vi "PumpGilsonGFV.vi"(8 "error in (no error)":errorcluster, 10 "?":T1=enum."Disable Pump", 11 "Variant in":variant) -> (0 "error out":errorcluster, 3 "Variant Out":variant)   [LabVIEW 2013]
doc: "Use this template to build a VI to use as a subVI."
uses:
  General TypeDefs/PumpGilson.ctl
  <vilib>/DAQmx/create/channels.llb/DAQmx Create Channel (DO-Digital Output).vi
  <vilib>/DAQmx/create/channels.llb/DAQmx Create Channel (AO-Voltage-Basic).vi
  <vilib>/DAQmx/write.llb/DAQmx Write (Digital 1D Bool NChan 1Samp 1Line).vi
  <vilib>/DAQmx/write.llb/DAQmx Write (Analog DBL 1Chan 1Samp).vi
  General TypeDefs/PumpGilsonEnum.ctl
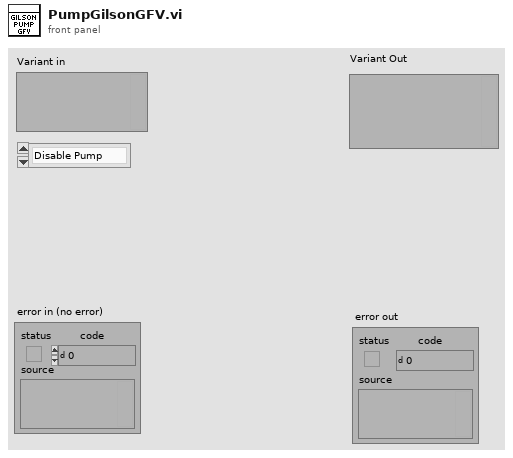
[diagram p1: front panel]
types:
  T1 = typedef "PumpGilsonEnum.ctl" = enum16{"Insert Measuremets Parameters", "Disable Pump", "Enable Pump", "SetPumpState", "SetPumpSpeed", "SetPumpDirection", "GetPumpParameters", "GetCommunicationParameters", "UpdatePumpUI", "ReadFromConfigurationFile", "Init"}
  T2 = typedef "PumpGilson.ctl" = cluster{"Pump Speed Port (analog 0-5 volts)":tag, "Pump State(line 0):Direction(line 1) (TTL output)":tag, "Pump Speed (0-5)":dbl, "Pumping Direction (pull/push)":bool, "Pump State (On/Off)":bool, "Gilson Pump Enabled(On/Off)":bool, "ON time before Acquire (sec)":dbl, "OFF time before Acquire (sec)":dbl}
  T3 = cluster{"ON time before Acquire (sec)":dbl, "OFF time before Acquire (sec)":dbl}
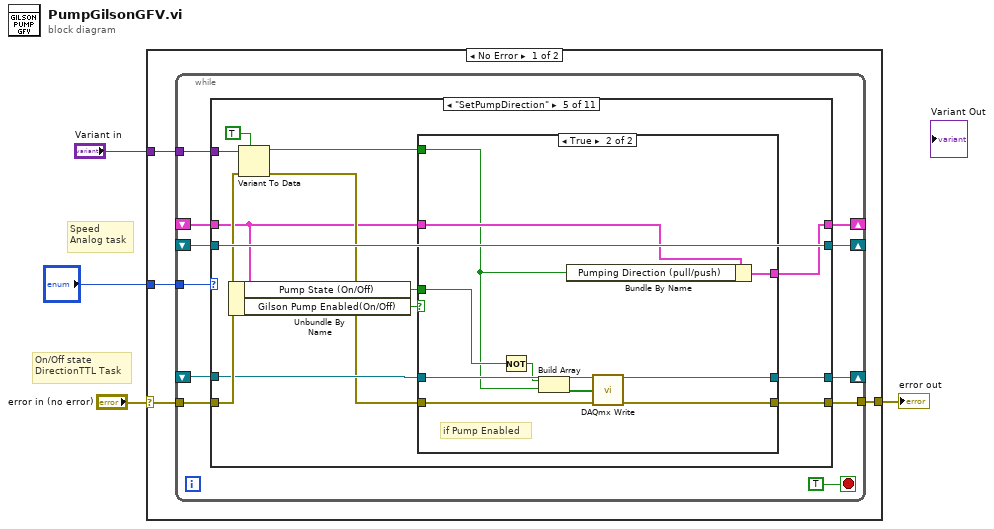
[diagram p0: block diagram]
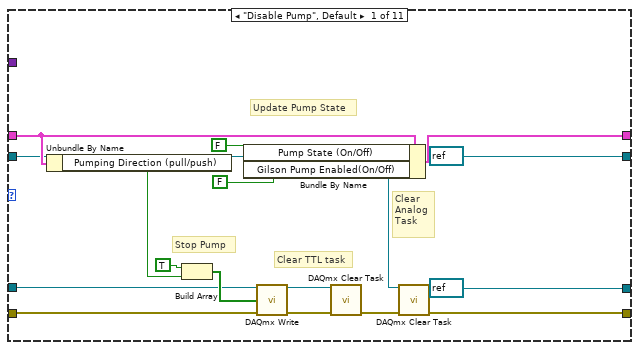
[diagram p2: hidden frame]
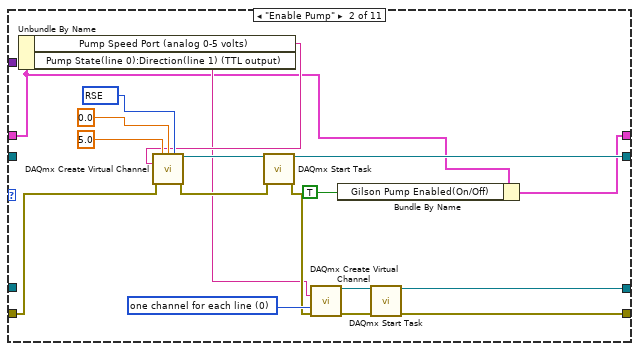
[diagram p3: hidden frame]
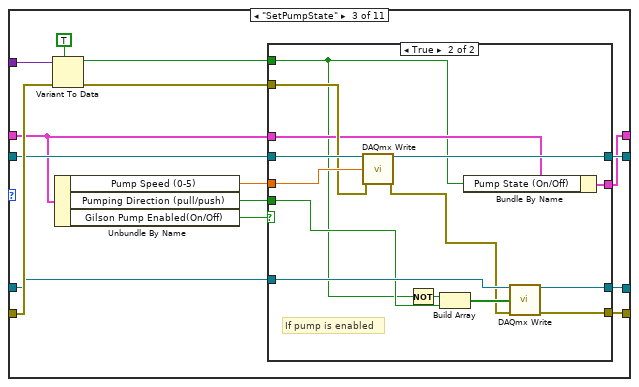
[diagram p4: hidden frame]
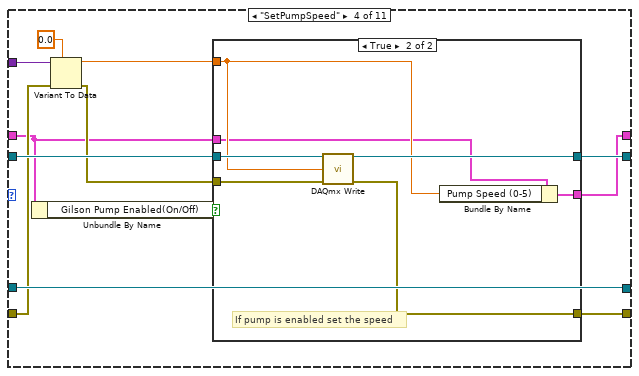
[diagram p6: hidden frame]
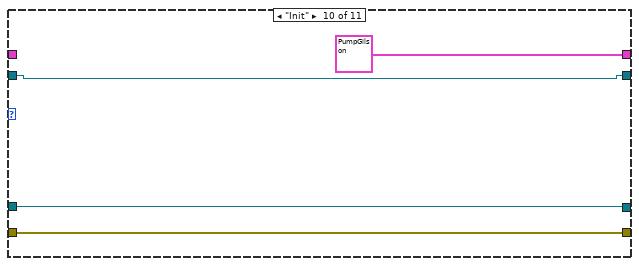
[diagram p13: hidden frame]
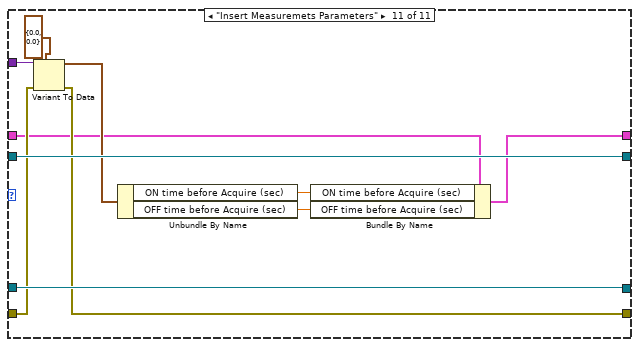
[diagram p14: hidden frame]
diagram:
  # "On/Off state\nDirectionTTL Task"
  # "Speed\nAnalog task"
  n1 = case shown="No Error" "error in (no error)" {
    selector: "error in (no error)" -> [w7 w166]
    tunnel: [w6 w166] -> w3
    tunnel: "?" -> [w8 _]
    tunnel: "Variant in" -> [w5 _]
    frame No Error {
      n2 = while {
        tunnel: w8 -> [w18]
        shift-right: [w17] -> _
        shift-left: _ -> [w14]
        tunnel: w7 -> [w16]
        tunnel: [w15] -> w6
        tunnel: w5 -> [w13]
        shift-right: [w12] -> _
        shift-left: _ -> [w9]
        shift-right: [w11] -> _
        shift-left: _ -> [w10]
        stop <- TRUE stop-if-true
        n3 = case shown="\"SetPumpDirection\"" w18 {
          tunnel: [w26 w36 w56 w93 w113 w138 w142 w146 w150 T2 {"Pump Speed Port (analog 0-5 volts)"="Gilson_Pump_IO/ao0", "Pump State(line 0):Direction(line 1) (TTL output)"="Gilson_Pump_IO/port0/line0:1", "Pump Speed (0-5)"=2.5, "Pumping Direction (pull/push)"=FALSE, "Pump State (On/Off)"=FALSE, "Gilson Pump Enabled(On/Off)"=FALSE, "ON time before Acquire (sec)"=0.0, "OFF time before Acquire (sec)"=0.0} ("PumpGilsonData") w155] -> w17
          tunnel: w16 -> [w30 w45 w68 w94 w119 w137 w141 w145 w149 w153 w162]
          tunnel: [w24 w43 w63 w89 w115 w137 w141 w145 w149 w153 w161] -> w15
          tunnel: w14 -> [w28 w37 w57 w88 w112 w138 w142 w146 w150 _ w156]
          tunnel: w13 -> [_ _ w67 w95 w120 _ _ _ _ _ w163]
          tunnel: [refnum<k21> refnum ("task out") w41 w59 w96 w121 w135 w139 w143 w147 w151 w165] -> w12
          tunnel: [refnum<k21> refnum ("task out") w40 w64 w98 w117 w136 w140 w144 w148 w152 w164] -> w11
          tunnel: w10 -> [w31 _ w65 w98 w118 w136 w140 w144 w148 w152 w164]
          tunnel: w9 -> [w23 _ w60 w97 w121 w135 w139 w143 w147 w151 w165]
          frame "Disable Pump", Default {
            # "Update Pump State"
            # "Stop Pump"
            # "Clear \nAnalog\nTask"
            # "Clear TTL task"
            n4 = Unbundle By Name(w28) -> ("Pumping Direction (pull/push)"=w29:bool)
            n5 = Build Array(TRUE ("element"), w29) -> (w33:bool[])
            n6 = Bundle By Name(cluster=w28, "Pump State (On/Off)"=FALSE, "Gilson Pump Enabled(On/Off)"=FALSE ("Enable Gilson Pump")) -> (w26:T2)
            n7 = call-poly <vilib>:"DAQmx Write.vi"("task/channels in"=w31, "data"=w33, "error in"=w30) -> ("task out"=w35:refnum<k21>, "error out"=w34:errorcluster)  [unwired: 10 in, 1 out]
            n8 = call <vilib>:"DAQmx Clear Task.vi"("task in"=w35, "error in"=w34) -> ("error out"=w25:errorcluster)  [unwired: 13 in]
            n9 = call <vilib>:"DAQmx Clear Task.vi"("task in"=w23, "error in"=w25) -> ("error out"=w24:errorcluster)  [unwired: 13 in]
          }
          frame "Enable Pump" {
            w46 = 0 items=["one channel for each line", "one channel for all lines"] ("line grouping")
            w51 = 10083 items=["Default"=-1, "RSE"=10083, "Differential"=10106, "Pseudodifferential"=12529] ("output terminal configuration")
            n10 = Unbundle By Name(w37) -> ("Pump Speed Port (analog 0-5 volts)"=w42:tag, "Pump State(line 0):Direction(line 1) (TTL output)"=w39:tag)
            n11 = call-poly <vilib>:"DAQmx Create Virtual Channel.vi"("maximum value"=5.0 ("minimum value"), "minimum value"=0.0, "output terminal configuration"=w51, "physical channels"=w42, "error in"=w45) -> ("task out"=w50:refnum<k21>, "error out"=w49:errorcluster)  [unwired: 9 in]
            n12 = call <vilib>:"DAQmx Start Task.vi"("task/channels in"=w50, "error in"=w49) -> ("task out"=w41:refnum<k21>, "error out"=w44:errorcluster)  [unwired: 12 in]
            n13 = call-poly <vilib>:"DAQmx Create Virtual Channel.vi"("lines"=w39, "line grouping"=w46, "error in"=w44) -> ("task out"=w47:refnum<k21>, "error out"=w48:errorcluster)  [unwired: 11 in]
            n14 = Bundle By Name(cluster=w37, "Gilson Pump Enabled(On/Off)"=TRUE ("Enable Gilson Pump")) -> (w36:T2)
            n15 = call <vilib>:"DAQmx Start Task.vi"("task/channels in"=w47, "error in"=w48) -> ("task out"=w40:refnum<k21>, "error out"=w43:errorcluster)  [unwired: 12 in]
          }
          frame "SetPumpState" {
            n16 = Variant To Data(error in=w68, type=TRUE ("Enable Gilson Pump"), Variant=w67) -> (data=w55:bool, error out=w58:errorcluster)
            n17 = Unbundle By Name(w57) -> ("Pump Speed (0-5)"=w61:dbl, "Pumping Direction (pull/push)"=w62:bool, "Gilson Pump Enabled(On/Off)"=w54:bool)
            n18 = case shown="True" w54 {
              tunnel: w65 -> [w69 w84]
              tunnel: [w69 w83] -> w64
              tunnel: [w70 w82] -> w63
              tunnel: w62 -> [_ w81]
              tunnel: w61 -> [_ w80]
              tunnel: w60 -> [w72 w79]
              tunnel: [w72 w78] -> w59
              tunnel: w58 -> [w70 w77]
              tunnel: w57 -> [w71 w75]
              tunnel: [w71 w74] -> w56
              tunnel: w55 -> [_ w73]
              frame False {
              }
              frame True {
                # "If pump is enabled"
                n19 = call-poly <vilib>:"DAQmx Write.vi"("task/channels in"=w79, "data"=w80, "error in"=w77) -> ("task out"=w78:refnum<k21>, "error out"=w76:errorcluster)  [unwired: 10 in, 1 out]
                n20 = Not(x=w73) -> (.not. x?=w85:bool)
                n21 = Build Array(w85, w81) -> (w86:bool[])
                n22 = Bundle By Name(cluster=w75, "Pump State (On/Off)"=w73) -> (w74:T2)
                n23 = call-poly <vilib>:"DAQmx Write.vi"("task/channels in"=w84, "data"=w86, "error in"=w76) -> ("task out"=w83:refnum<k21>, "error out"=w82:errorcluster)  [unwired: 10 in, 1 out]
              }
            }
          }
          frame "SetPumpSpeed" {
            n24 = Unbundle By Name(w88) -> ("Gilson Pump Enabled(On/Off)"=w87:bool)
            n25 = Variant To Data(error in=w94, type=0.0 ("Pump Speed (0-5)"), Variant=w95) -> (data=w91:dbl, error out=w90:errorcluster)
            n26 = case shown="True" w87 {
              tunnel: w97 -> [w101 w108]
              tunnel: [w101 w107] -> w96
              tunnel: [w100 w106] -> w93
              tunnel: w91 -> [_ w105]
              tunnel: w90 -> [w99 w104]
              tunnel: [w99 w103] -> w89
              tunnel: w88 -> [w100 w102]
              frame False {
              }
              frame True {
                # "If pump is enabled set the speed"
                n27 = call-poly <vilib>:"DAQmx Write.vi"("task/channels in"=w108, "data"=w105, "error in"=w104) -> ("task out"=w107:refnum<k21>, "error out"=w103:errorcluster)  [unwired: 10 in, 1 out]
                n28 = Bundle By Name(cluster=w102, "Pump Speed (0-5)"=w105) -> (w106:T2)
              }
            }
          }
          frame "SetPumpDirection" {
            n29 = Unbundle By Name(w112) -> ("Pump State (On/Off)"=w111:bool, "Gilson Pump Enabled(On/Off)"=w109:bool)
            n30 = Variant To Data(error in=w119, type=TRUE ("Enable Gilson Pump"), Variant=w120) -> (data=w110:bool, error out=w116:errorcluster)
            n31 = case shown="True" w109 {
              tunnel: w118 -> [w123 w133]
              tunnel: [w123 w132] -> w117
              tunnel: w116 -> [w122 w131]
              tunnel: [w122 w130] -> w115
              tunnel: [w124 w129] -> w113
              tunnel: w112 -> [w124 w128]
              tunnel: w111 -> [_ w126]
              tunnel: w110 -> [_ w125]
              frame False {
              }
              frame True {
                # "if Pump Enabled"
                n32 = Not(x=w126) -> (.not. x?=w127:bool)
                n33 = Build Array(w127, w125) -> (w134:bool[])
                n34 = Bundle By Name(cluster=w128, "Pumping Direction (pull/push)"=w125) -> (w129:T2)
                n35 = call-poly <vilib>:"DAQmx Write.vi"("task/channels in"=w133, "data"=w134, "error in"=w131) -> ("task out"=w132:refnum<k21>, "error out"=w130:errorcluster)  [unwired: 10 in, 1 out]
              }
            }
          }
          frame "GetPumpParameters" {
          }
          frame "GetCommunicationParameters" {
          }
          frame "UpdatePumpUI" {
          }
          frame "ReadFromConfigurationFile" {
          }
          frame "Init" {
          }
          frame "Insert Measuremets Parameters" {
            n36 = Variant To Data(error in=w162, type=T3 {"ON time before Acquire (sec)"=0.0, "OFF time before Acquire (sec)"=0.0} ("output cluster"), Variant=w163) -> (data=w159:T3, error out=w161:errorcluster)
            n37 = Unbundle By Name(w159) -> ("ON time before Acquire (sec)"=w158:dbl, "OFF time before Acquire (sec)"=w157:dbl)
            n38 = Bundle By Name(cluster=w156, "ON time before Acquire (sec)"=w158, "OFF time before Acquire (sec)"=w157) -> (w155:T2)
          }
        }
      }
    }
    frame Error {
    }
  }
  "error out" <- w3
